vi "fir_test4.vi"() -> ()   [LabVIEW 2013]
uses:
  <vilib>/measure/maspectr.llb/Power Spectrum and PSD Export Mode.ctl
  <vilib>/measure/maspectr.llb/FFT Power Spectrum and PSD for 1 Chan.vi
  <vilib>/measure/NI_MABase.lvlib
  <vilib>/measure/NI_MAPro.lvlib
panel:
  out "double precision float 2":dbl[](array[numeric])
  out "double precision float":dbl[](array[numeric])
  out "Waveform Graph out":dbl[](graph)
  out "Power spectrum in":cluster{"f0":dbl, "df":dbl, "magnitude":dbl[]}(graph)
  out "Power spectrum":cluster{"f0":dbl, "df":dbl, "magnitude":dbl[]}(graph)
  out "Waveform Graph":dbl[](graph)
  out "# of Iterations":i32
  out "# of samples":i32
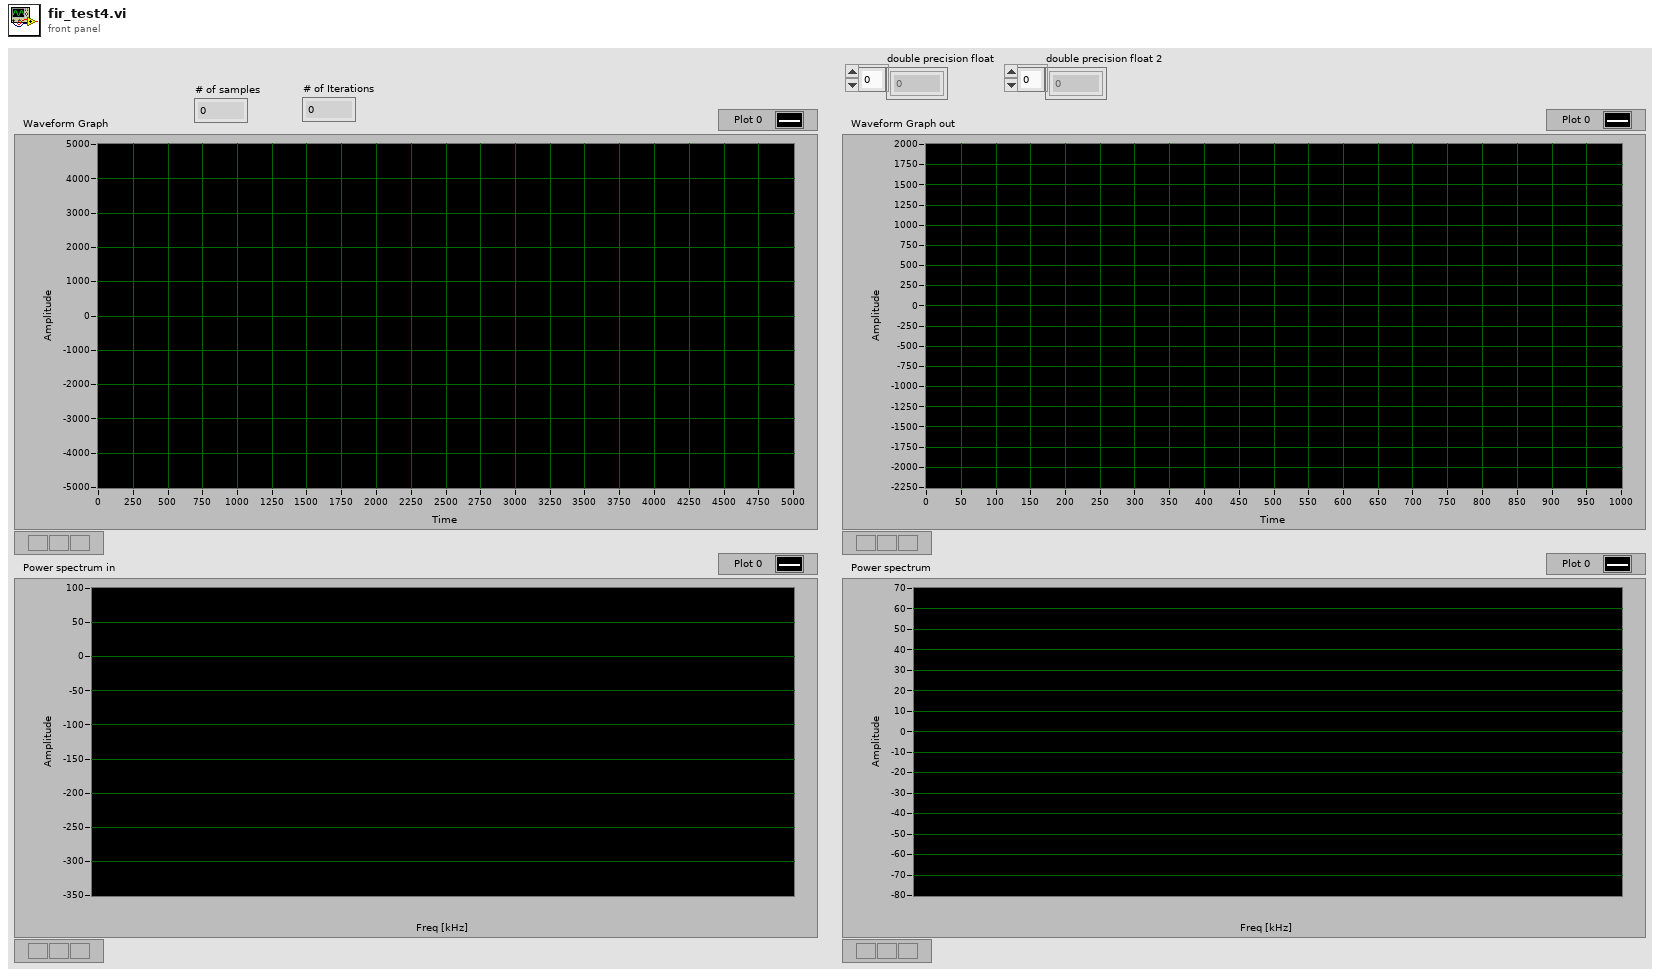
[diagram p1: front panel]
types:
  T1 = typedef "NI_MAPro.lvlib/Power Spectrum and PSD Export Mode.ctl" = u16
  T2 = cluster{"frequency":dbl, "amplitude":dbl, "phase":dbl}[]
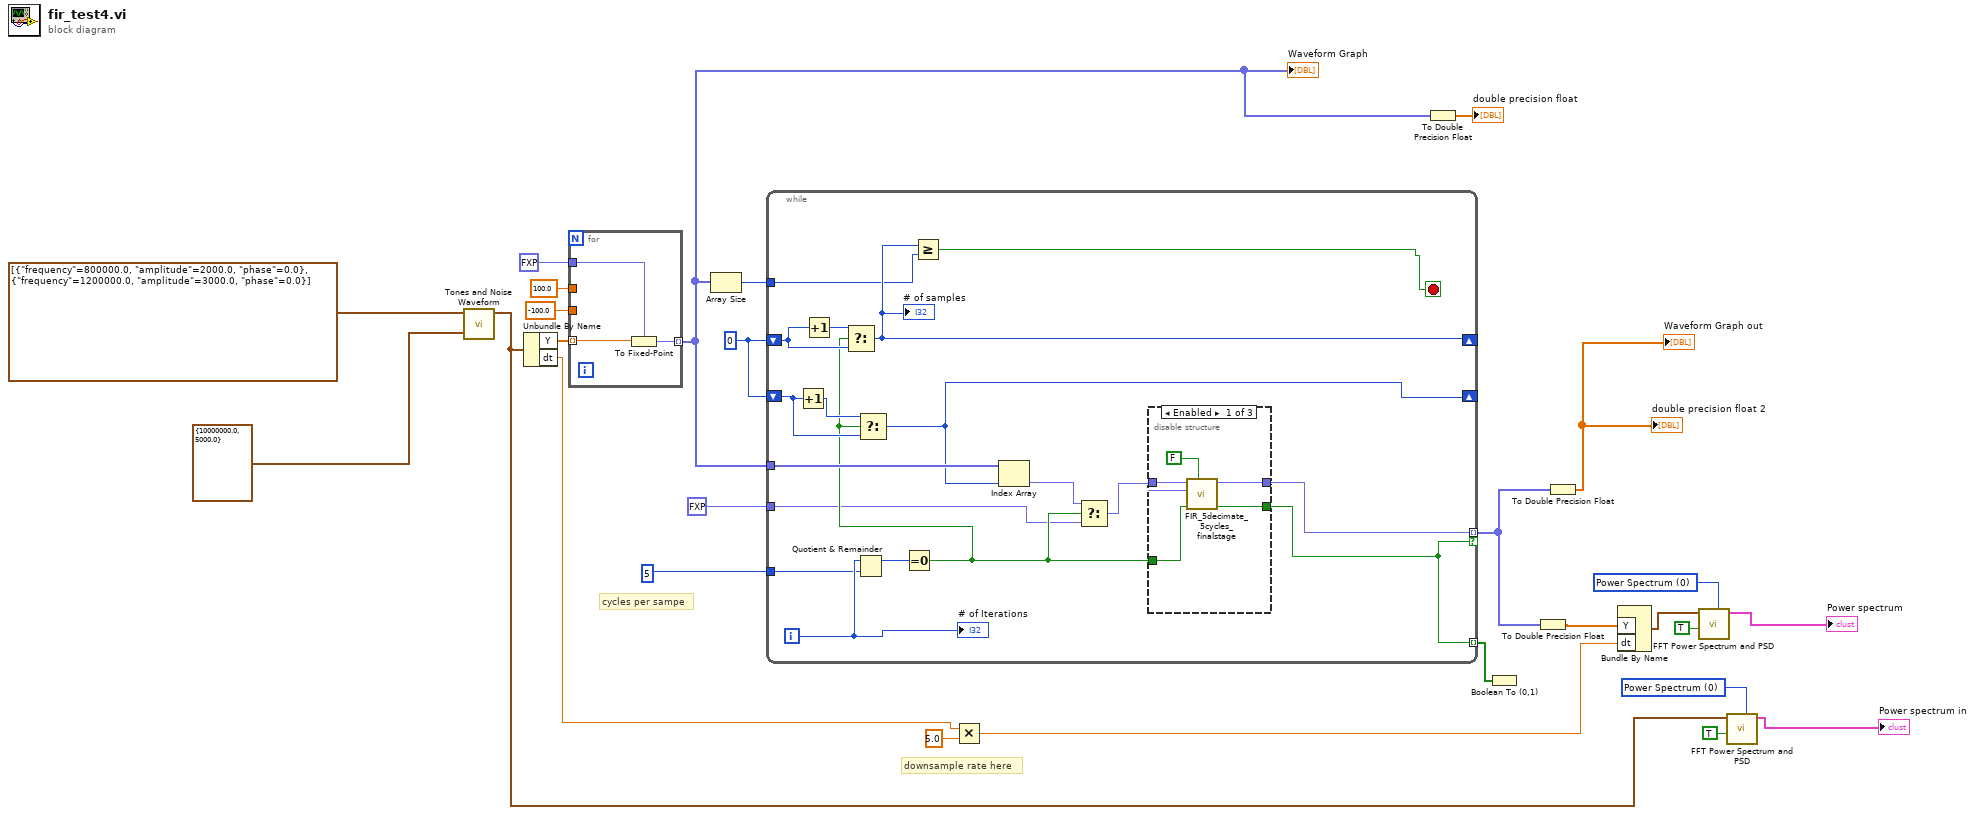
[diagram p0: block diagram]
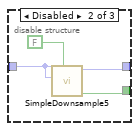
[diagram p2: hidden frame]
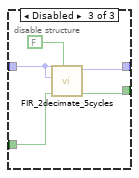
[diagram p3: hidden frame]
diagram:
  w12 = T1 0 items=["Power Spectrum", "Power Spectral Density"] ("export mode")
  w21 = T1 0 items=["Power Spectrum", "Power Spectral Density"] ("export mode")
  w23 = 0 ("samples")
  # "cycles per sampe"
  # "downsample rate here"
  n1 = call <vilib>:"Tones and Noise Waveform.vi"("sampling info"=cluster{"Fs":dbl, "#s":dbl} {"Fs"=10000000.0, "#s"=5000.0}, "tones"=T2 [{"frequency"=800000.0, "amplitude"=2000.0, "phase"=0.0}, {"frequency"=1200000.0, "amplitude"=3000.0, "phase"=0.0}]) -> ("signal out"=w11:waveform(dbl))  [unwired: 8 in, 1 out]
  n2 = Unbundle By Name(w11) -> ("Y"=w19:dbl[], "dt"=w18:dbl)
  n3 = for {
    tunnel: w19 -> [w28] mode=indexing
    tunnel: fxp<+/-,16,14> 0.0 ("fixed-point type") -> [w30]
    tunnel: [w29] -> w4 mode=indexing
    tunnel: 100.0 -> [_]
    tunnel: -100.0 -> [_]
    n4 = To Fixed-Point(fixed-point type=w30, number=w28) -> (fixed-point=w29:fxp<+/-,16,14>)
  }
  "Waveform Graph" <- w4
  n5 = Array Size(array=w4) -> (size(s)=w24:i32)
  n6 = while {
    tunnel: w4 -> [w48]
    shift-right: [w40] -> _
    shift-left: w23 -> [w46]
    shift-right: [w43] -> _
    shift-left: w23 -> [w44]
    tunnel: [w39] -> w9 mode=indexing if=w31
    tunnel: w24 -> [w41]
    tunnel: 5 ("samples") -> [w37]
    tunnel: fxp<+/-,16,14> 0.0 ("fixed-point type") -> [w33]
    tunnel: [w31] -> w2 mode=indexing
    i -> [w38]
    stop <- w42 stop-if-true
    n7 = Increment(x=w46) -> (x+1=w47:i32)
    n8 = Increment(x=w44) -> (x+1=w45:i32)
    n9 = Quotient & Remainder(x=w38, y=w37) -> (x-y*floor(x/y)=w36:i32)  [unwired: 1 out]
    n10 = Equal To 0?(x=w36) -> (x = 0?=w35:bool)
    n11 = Select(t=w45, s=w35, f=w44) -> (s? t:f=w43:i32)
    "# of samples" <- w43
    n12 = Select(t=w47, s=w35, f=w46) -> (s? t:f=w40:i32)
    n13 = Greater Or Equal?(x=w43, y=w41) -> (x >= y?=w42:bool)
    n14 = Index Array(array=w48, index=w40) -> (element=w34:fxp<+/-,16,14>)
    n15 = Select(t=w34, s=w35, f=w33) -> (s? t:f=w32:fxp<+/-,16,14>)
    n16 = disable-structure shown="Enabled" {
      disable-tunnel: [w52 w57 w62] -> w39
      disable-tunnel: [w51 w56 w61] -> w31
      disable-tunnel: w35 -> [w50 _ w60]
      disable-tunnel: w32 -> [w49 w54 w58]
      frame Enabled {
        n17 = call "FIR_5decimate_5cycles_finalstage.vi"("reset"=FALSE, "valid in"=w50, "Q in"=w49, "I in"=w49) -> ("valid out"=w51:bool, "I out"=w52:fxp<+/-,16,14>)  [unwired: 4 in, 2 out]
      }
      frame Disabled {
        n18 = call "SimpleDownsample5.vi"("reset"=FALSE, "Data in 1"=w54, "Data in 0"=w54) -> ("data valid"=w56:bool, "Data out"=w57:fxp<+/-,16,14>)  [unwired: 7 in]
      }
      frame Disabled {
        n19 = call "FIR_2decimate_5cycles.vi"("reset"=FALSE, "valid in"=w60, "Q in"=w58, "I in"=w58) -> ("valid out"=w61:bool, "I out"=w62:fxp<+/-,16,14>)  [unwired: 4 in, 2 out]
      }
    }
    "# of Iterations" <- w38
  }
  n20 = Multiply(x=w18, y=5.0) -> (x*y=w16:dbl)
  n21 = To Double Precision Float(number=w4) -> (double precision float=→"double precision float":dbl[])
  n22 = Boolean To (0,1)(Boolean=w2) -> ()  [unwired: 1 out]
  n23 = To Double Precision Float(number=w9) -> (double precision float=w14:dbl[])
  n24 = To Double Precision Float(number=w9) -> (double precision float=→"Waveform Graph out" →"double precision float 2":dbl[])
  n25 = Bundle By Name("Y"=w14, "dt"=w16) -> (w22:waveform(dbl))  [unwired: 1 in]
  n26 = call-poly <vilib>:"FFT Power Spectrum and PSD.vi"("export mode"=w21, "dB On (F)"=TRUE, "time signal"=w22) -> ("Power Spectrum / PSD"=→"Power spectrum":cluster{"f0":dbl, "df":dbl, "magnitude":dbl[]})  [unwired: 5 in, 3 out]
  n27 = call-poly <vilib>:"FFT Power Spectrum and PSD.vi"("export mode"=w12, "dB On (F)"=TRUE, "time signal"=w11) -> ("Power Spectrum / PSD"=→"Power spectrum in":cluster{"f0":dbl, "df":dbl, "magnitude":dbl[]})  [unwired: 5 in, 3 out]
